vi "FdxCmdTMSetRequestNumberCvi.vi"(8 "error in":errorcluster, 9 "RequestNumber":u16, 10 "TMHandle":u32, 11 "InstrumentHandle":u32) -> (0 "error out":errorcluster, 2 "TMHandleOut":u32, 3 "InstrumentHandle":u32)   [LabVIEW 2020, in "AIM664LV.lvlib"]
doc: "This function is used to set the Time Manager request number on the next Time Manager Iteration. The Request Number will continue incrementing by one from the set value with each subsequent Time Manager Iteration."
uses:
  AIM664LV.lvlib
  AFDX_LibraryAdmin/FdxGlobalDllPath.vi
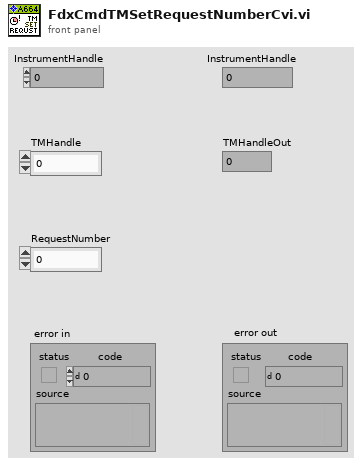
[diagram p1: front panel]
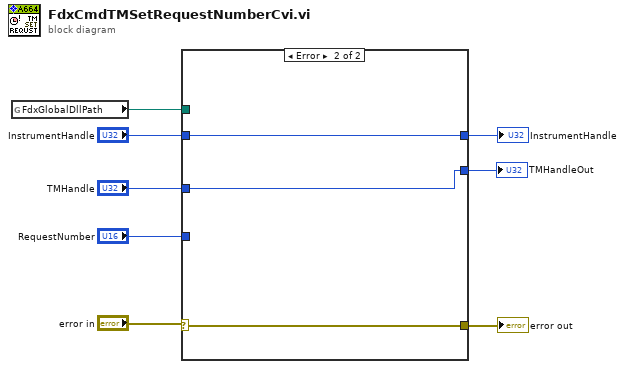
[diagram p0: block diagram]
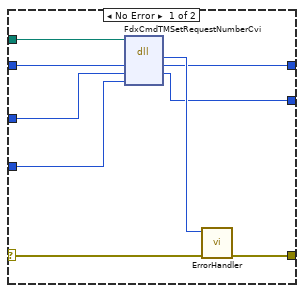
[diagram p2: hidden frame]
diagram:
  n1 = global read "FdxGlobalDllPath.vi" "FdxGlobalDllPath"() -> (w6:path)
  n2 = case shown="Error" "error in" {
    selector: "error in" -> [w16 w20]
    tunnel: [w17 w20] -> w8
    tunnel: w6 -> [w14 _]
    tunnel: "InstrumentHandle" -> [w13 w19]
    tunnel: [w12 w19] -> w4
    tunnel: "TMHandle" -> [w11 w18]
    tunnel: "RequestNumber" -> [w10 _]
    tunnel: [w9 w18] -> w1
    frame No Error {
      n3 = dll-call lib="aim_fdx.19.dll" fn="FdxCmdTMSetRequestNumberCvi" label="TMSetRequestNumberCvi"(path in=w14, "InstrumentHandle"=w13, "TMHandle"=w11, "RequestNumber"=w10) -> ("status"=w15:i32, "InstrumentHandle"=w12:u32, "TMHandle"=w9:u32)  [unwired: 3 in, 2 out]
      n4 = call "ErrorHandler.vi"("error in"=w16, "AIM Error"=w15) -> ("error out"=w17:errorcluster)  [unwired: 9 in]
    }
    frame Error {
    }
  }
  "error out" <- w8
  "InstrumentHandle" <- w4
  "TMHandleOut" <- w1
